vi "Emerson 5700 Example.vi"(8 "Error In":errorcluster, 10 "Remote Port":u16=502, 11 "Remote IP Address":string="10.2.0.49") -> (0 "Error Out":errorcluster, 3 "Emerson Flow Meter Data Output":T2={"Mass Flow Rate (Scaled Integer)"=0, "Density (Scaled Integer)"=8, "Temperature (Scaled Integer)"=114, "Volume Flow Rate (Scaled Integer)"=0, "Totalizer 1 (Scaled Integer)"=5, "Totalizer 2 (Scaled Integer)"=0, "Transmitter Software Rev"=14, "Flow Direction"="Forward", "Mass Flow Units"="lb/min", "Density Units"="lb/US Gal", "Temperature Units"="°F", "Volume Flow Units"="US GPM", "Pressure Units"="PSI", "Mass Total Units"="lbs", "Volume Total Units"="US Gallon", "Inventory 1 (Scaled Integer)"=5, "Inventory 2 (Scaled Integer)"=0, "Mass Flow Rate"=0.0, "Density"=8.2493896484375, "Temperature"=114.62187957763672, "Volume Flow Rate"=0.0, "Pressure (Scaled Integer)"=0, "Current Value Totalizer 1 (Pounds per draw)"=5.467781066894531, "Current Value Totalizer 2 (Gallons per draw)"=0.6632421612739563, "Current Value Inventory 1 (Pounds Total)"=5.467781066894531, "Current Value Inventory 2 (Gallons Total)"=0.6632421612739563, "Drive Gain"=7.360586643218994, "Raw Tube Frequency (Hz)"=151.36962890625, "Dynamic Viscosity (Centipoise)"=0.0, "Kinematic Viscosity (Centistokes)"=0.0, "Hot Gallons (Calculated Gallons)"=0.0, "Hot Flow Rate (Calculated GPM)"=0.0, "Hot Gallons Inventory (Gallons)"=0.0, "Hot Flow Rate (Laurel)"=0.0, "Hot Gallons (Laurel)"=0.0})   [LabVIEW 2019]
uses:
  Type Definitions/Emerson 5700 Data.ctl
  Type Definitions/Emerson 5700 Modbus Write Coils.ctl
  <vilib>/NI/Modbus Library/API/Master/Modbus Master.lvclass
  <vilib>/NI/Modbus Library/API/Wrapper/Create TCP Master.vi
  <vilib>/NI/Modbus Library/API/Wrapper/API Main.lvlib
panel:
  in  "address":string
  in  "Start/Stop Inventory 2.":T1=368 items=["Start/Stop Inventory 1"=367, "Start/Stop Inventory 2"=368, "Start/Stop all Totalizers and Inventories"=2, "Reset all Totalizers"=3, "Reset all Inventories"=4, "Reset Totalizer 1"=56, "Reset Totalizer 2"=57]
  in  "Start/Stop Inventory 1.":T1=367 items=["Start/Stop Inventory 1"=367, "Start/Stop Inventory 2"=368, "Start/Stop all Totalizers and Inventories"=2, "Reset all Totalizers"=3, "Reset all Inventories"=4, "Reset Totalizer 1"=56, "Reset Totalizer 2"=57]
  in  "Start/Stop Inventory 1":bool
  in  "Start/Stop Inventory 2":bool
  in  "Start/Stop all Totalizers and Inventories":bool
  in  "Reset all Totalizers":bool
  in  "Reset all Inventories":bool
  in  "Start/Stop all Totalizers and Inventories.":T1=2 items=["Start/Stop Inventory 1"=367, "Start/Stop Inventory 2"=368, "Start/Stop all Totalizers and Inventories"=2, "Reset all Totalizers"=3, "Reset all Inventories"=4, "Reset Totalizer 1"=56, "Reset Totalizer 2"=57]
  in  "Reset all Totalizers.":T1=3 items=["Start/Stop Inventory 1"=367, "Start/Stop Inventory 2"=368, "Start/Stop all Totalizers and Inventories"=2, "Reset all Totalizers"=3, "Reset all Inventories"=4, "Reset Totalizer 1"=56, "Reset Totalizer 2"=57]
  in  "Reset all Inventories.":T1=4 items=["Start/Stop Inventory 1"=367, "Start/Stop Inventory 2"=368, "Start/Stop all Totalizers and Inventories"=2, "Reset all Totalizers"=3, "Reset all Inventories"=4, "Reset Totalizer 1"=56, "Reset Totalizer 2"=57]
  in  "Reset Totalizer 2.":T1=57 items=["Start/Stop Inventory 1"=367, "Start/Stop Inventory 2"=368, "Start/Stop all Totalizers and Inventories"=2, "Reset all Totalizers"=3, "Reset all Inventories"=4, "Reset Totalizer 1"=56, "Reset Totalizer 2"=57]
  in  "Reset Totalizer 1.":T1=56 items=["Start/Stop Inventory 1"=367, "Start/Stop Inventory 2"=368, "Start/Stop all Totalizers and Inventories"=2, "Reset all Totalizers"=3, "Reset all Inventories"=4, "Reset Totalizer 1"=56, "Reset Totalizer 2"=57]
  in  "Reset Totalizer 2":bool
  in  "Reset Totalizer 1":bool
  in  "Emerson Flow Meter Data Input":T2
  # "Send Commands"
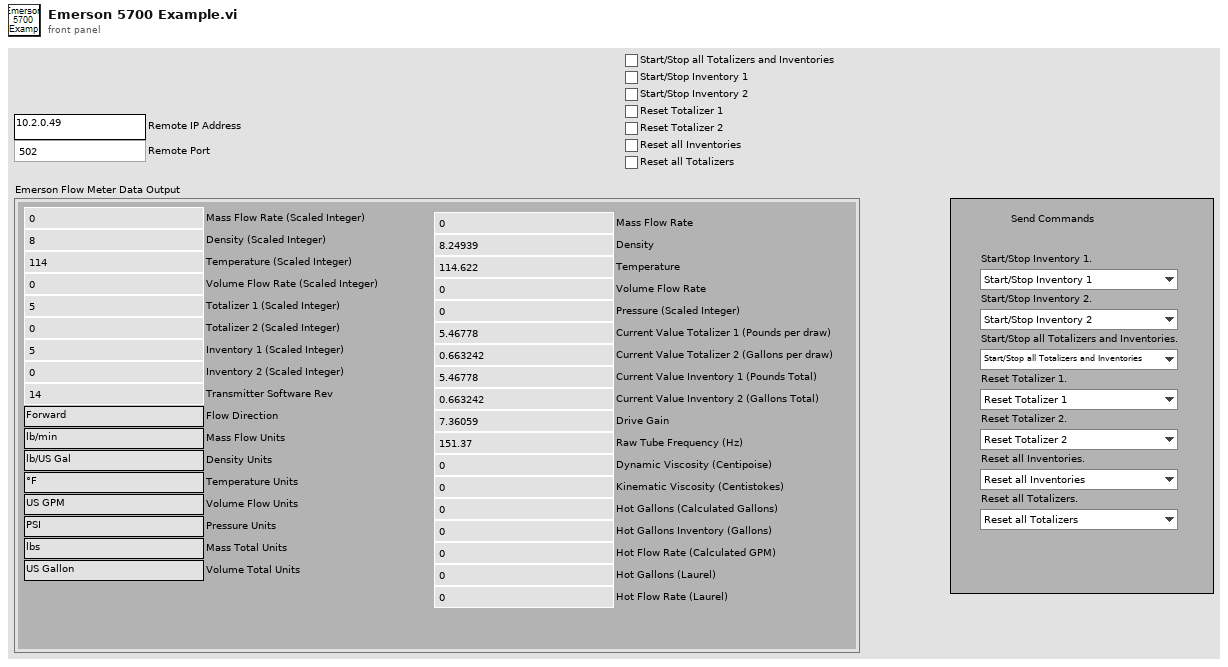
[diagram p1: front panel]
types:
  T1 = typedef "Emerson 5700 Modbus Write Coils.ctl" = u16
  T2 = typedef "Emerson 5700 Data.ctl" = cluster{"Mass Flow Rate (Scaled Integer)":u16, "Density (Scaled Integer)":u16, "Temperature (Scaled Integer)":u16, "Volume Flow Rate (Scaled Integer)":u16, "Totalizer 1 (Scaled Integer)":u16, "Totalizer 2 (Scaled Integer)":u16, "Transmitter Software Rev":u16, "Flow Direction":string, "Mass Flow Units":string, "Density Units":string, "Temperature Units":string, "Volume Flow Units":string, "Pressure Units":string, "Mass Total Units":string, "Volume Total Units":string, "Inventory 1 (Scaled Integer)":u16, "Inventory 2 (Scaled Integer)":u16, "Mass Flow Rate":dbl, "Density":dbl, "Temperature":dbl, "Volume Flow Rate":dbl, "Pressure (Scaled Integer)":u16, "Current Value Totalizer 1 (Pounds per draw)":dbl, "Current Value Totalizer 2 (Gallons per draw)":dbl, "Current Value Inventory 1 (Pounds Total)":dbl, "Current Value Inventory 2 (Gallons Total)":dbl, "Drive Gain":dbl, "Raw Tube Frequency (Hz)":dbl, "Dynamic Viscosity (Centipoise)":dbl, "Kinematic Viscosity (Centistokes)":dbl, "Hot Gallons (Calculated Gallons)":dbl, "Hot Flow Rate (Calculated GPM)":dbl, "Hot Gallons Inventory (Gallons)":dbl, "Hot Flow Rate (Laurel)":dbl, "Hot Gallons (Laurel)":dbl}
  T3 = enum32{"invalid app kind", "Development System", "Run Time System", "Student Edition", "Embedded LabVIEW", "Evaluation", "Custom"}
  T4 = enum32{"Invalid", "Standard", "Closed", "Hidden", "Minimized", "Maximized"}
  T5 = cluster{"Core":cluster{"Current VI Reference":refnum<vi>, "Close Panel on Exit?":bool}, "Remote IP Address":string, "Remote Port":u16, "TCP master instance":refnum<class "Modbus Master.lvclass">, "Emerson Flow Meter Data Input":T2}
  T6 = cluster{"Current VI Reference":refnum<vi>, "Close Panel on Exit?":bool}
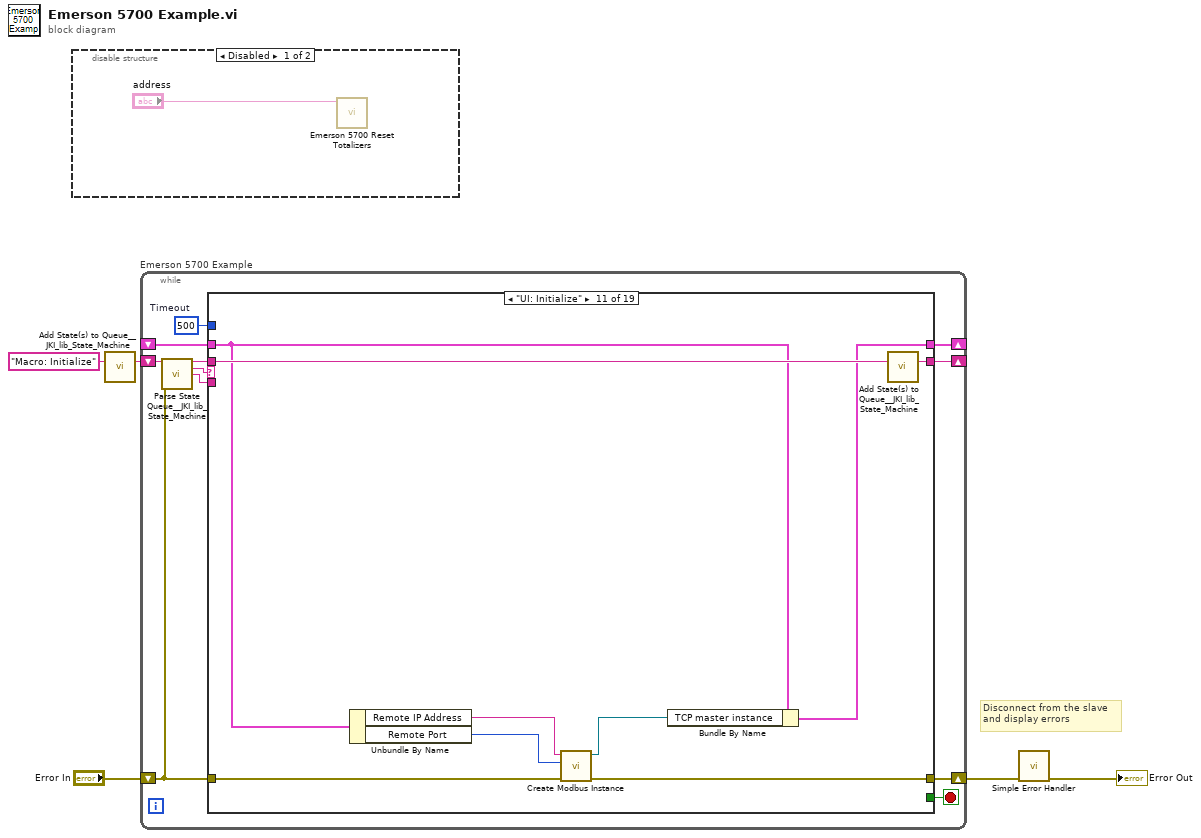
[diagram p0: block diagram]
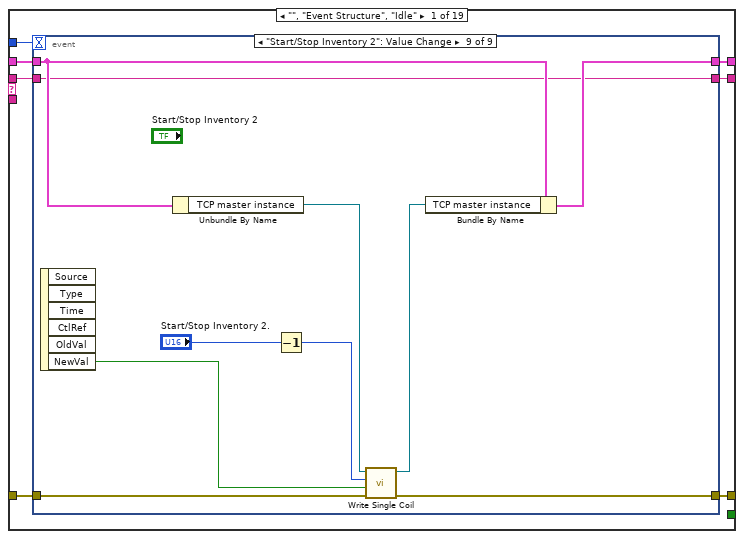
[diagram p3: hidden frame]
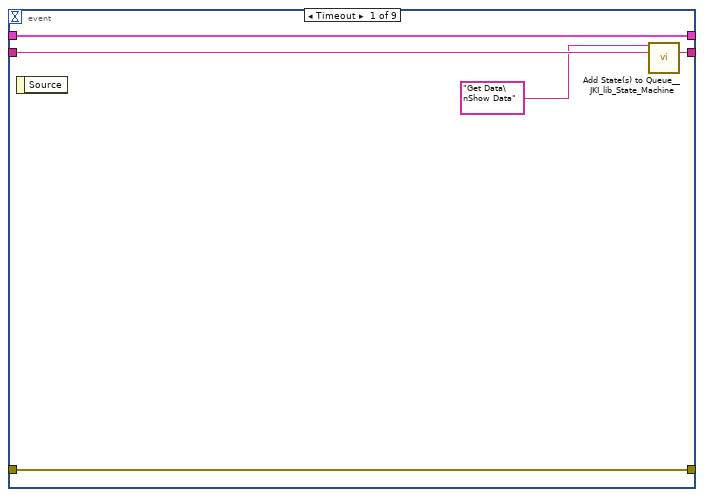
[diagram p4: hidden frame]
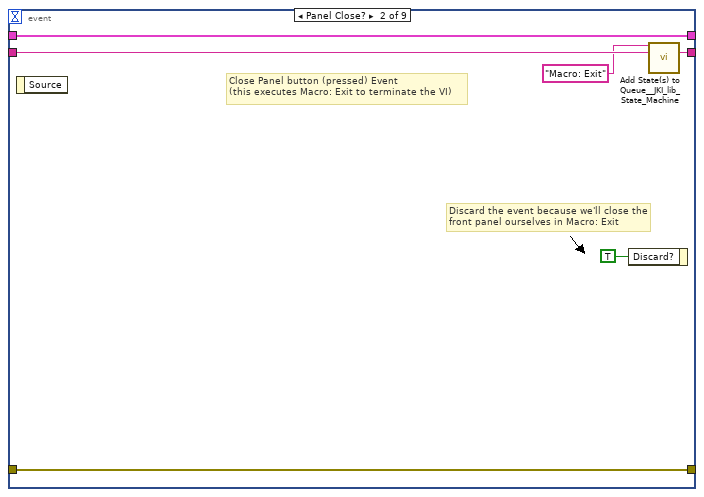
[diagram p5: hidden frame]
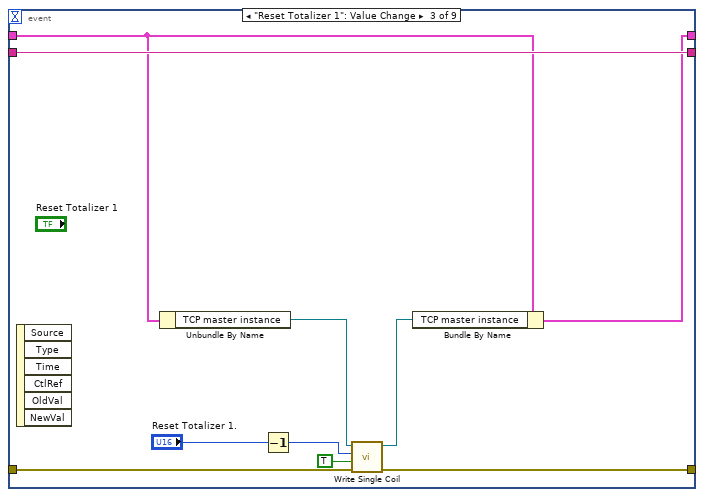
[diagram p6: hidden frame]
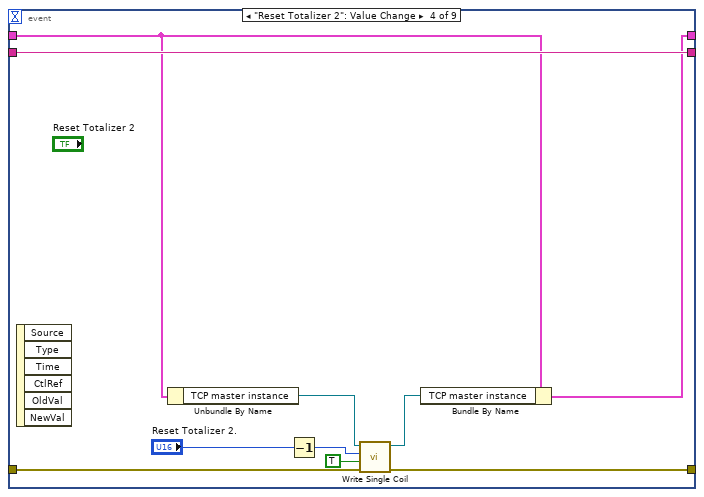
[diagram p7: hidden frame]
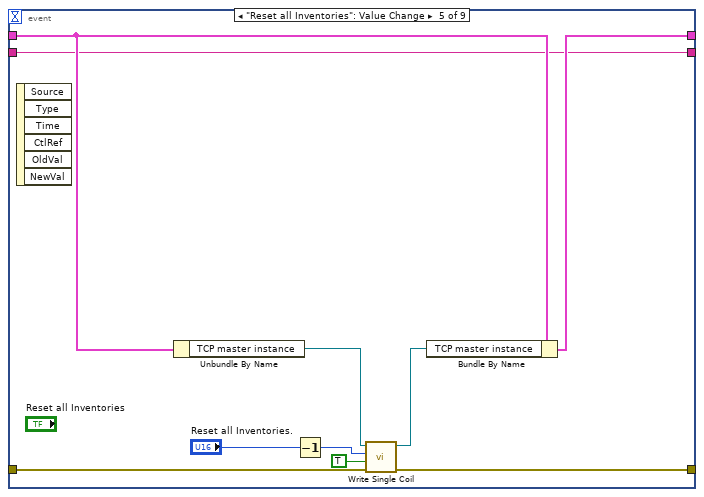
[diagram p8: hidden frame]
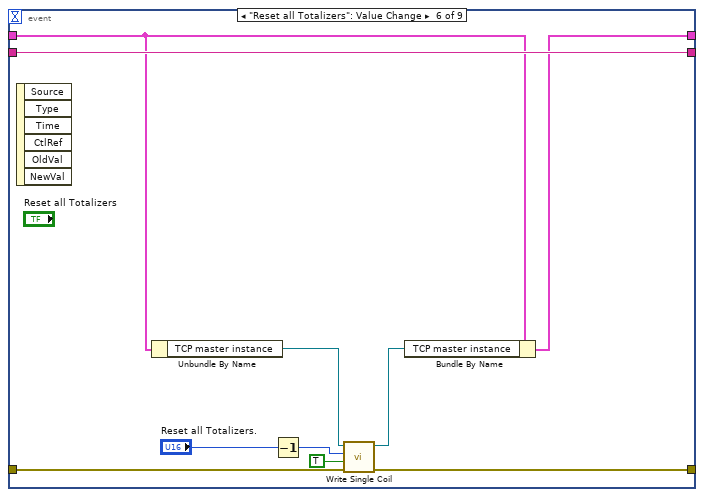
[diagram p9: hidden frame]
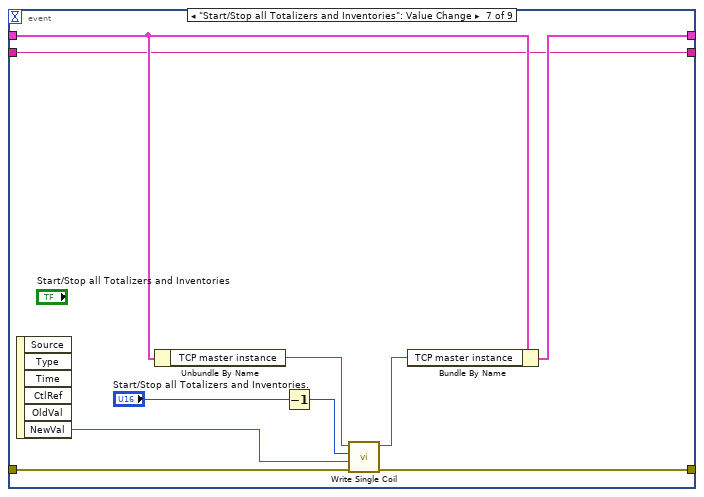
[diagram p10: hidden frame]
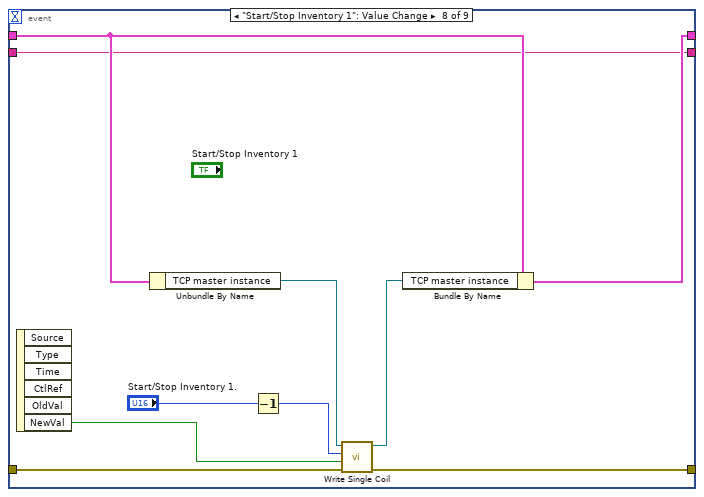
[diagram p11: hidden frame]
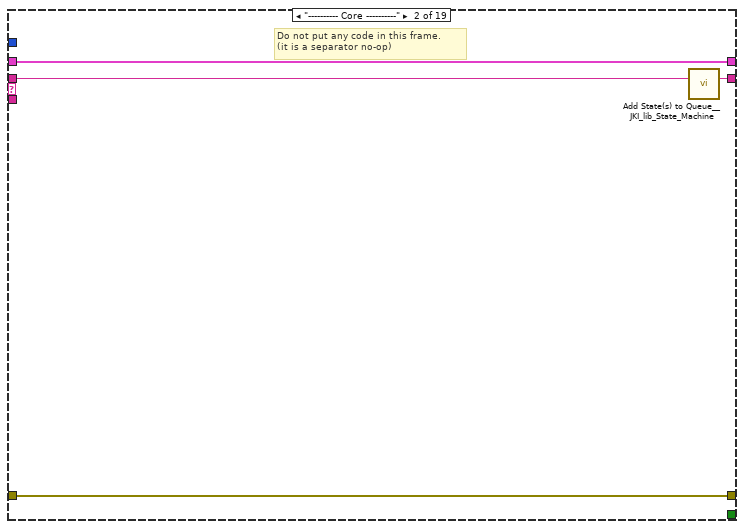
[diagram p12: hidden frame]
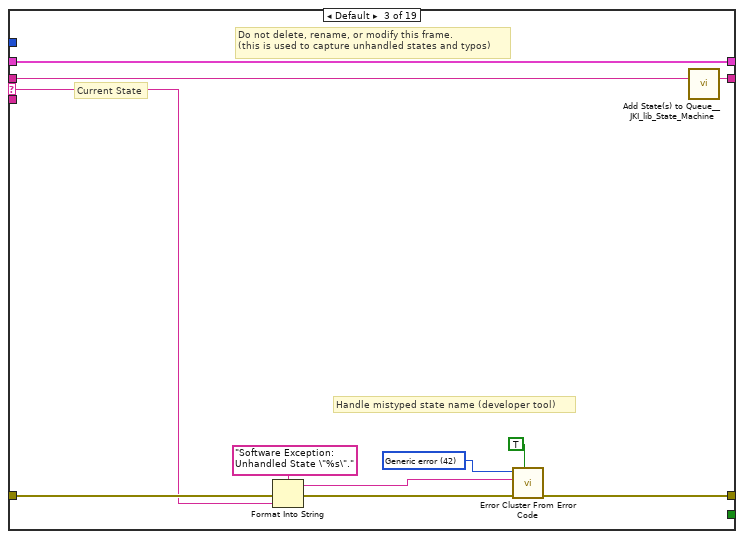
[diagram p13: hidden frame]
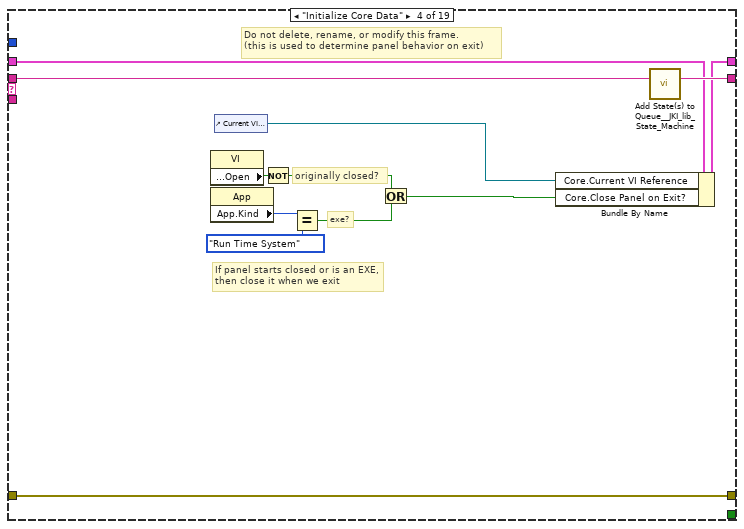
[diagram p14: hidden frame]
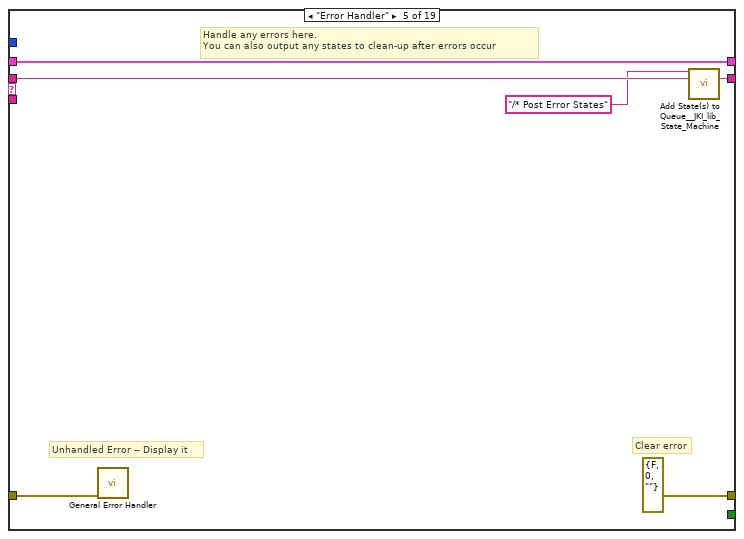
[diagram p15: hidden frame]
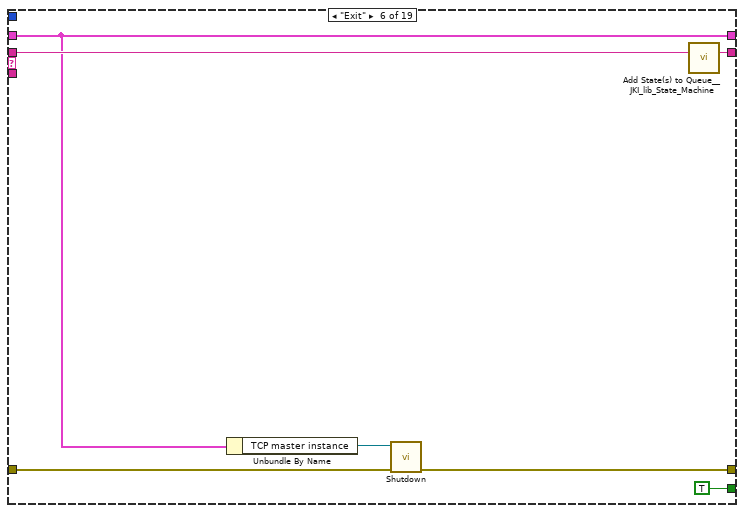
[diagram p16: hidden frame]
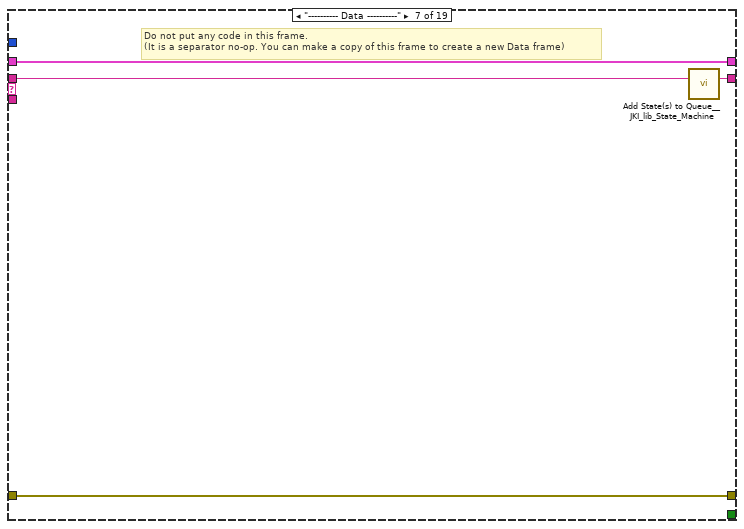
[diagram p17: hidden frame]
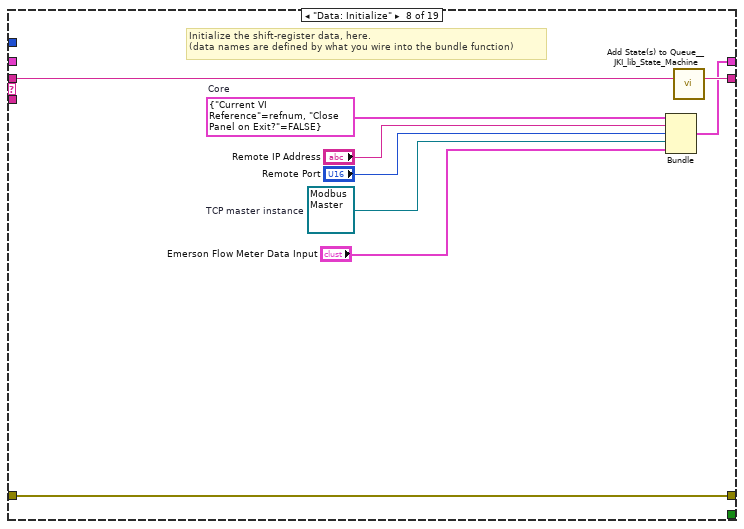
[diagram p18: hidden frame]
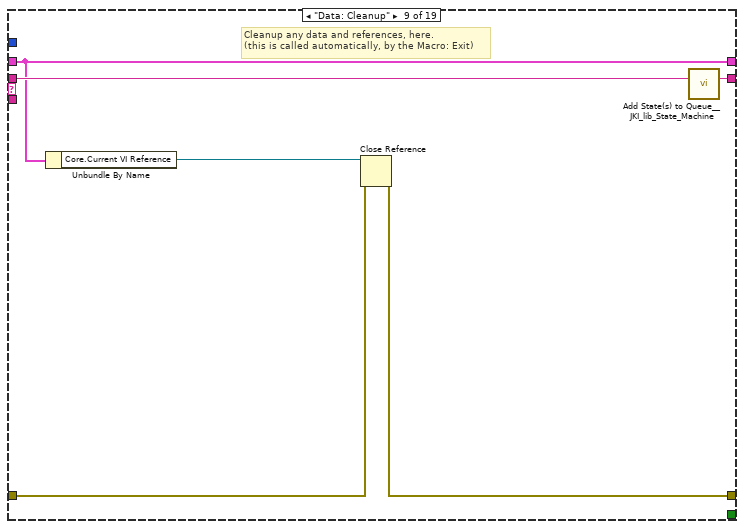
[diagram p19: hidden frame]
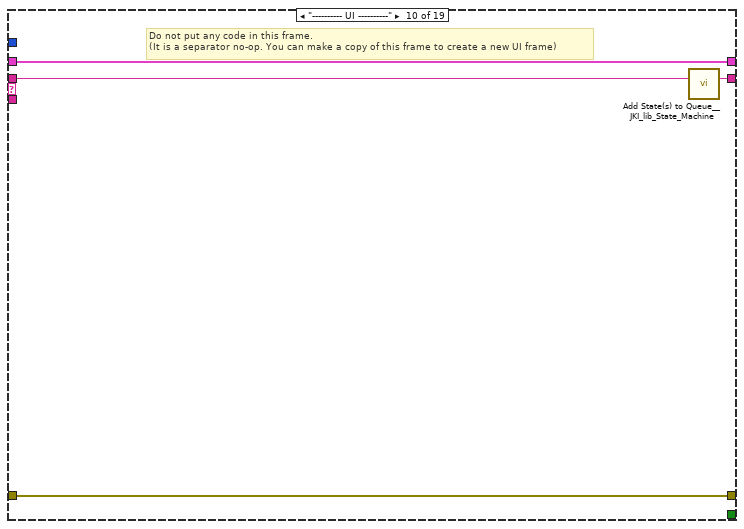
[diagram p20: hidden frame]
diagram:
  # "Disconnect from the slave\nand display errors"
  n1 = disable-structure shown="Disabled" {
    frame Disabled {
      n2 = call "Emerson 5700 Reset Totalizers.vi"("address"="address") -> ()  [unwired: 10 in, 1 out]
    }
    frame Enabled {
    }
  }
  n3 = call <vilib>:"Add State(s) to Queue__JKI_lib_State_Machine.vi"("State(s) in (\"\")"="Macro: Initialize") -> ("States Out"=w5:string)  [unwired: 14 in]
  n4 = while "Emerson 5700 Example" {
    shift-right: [w10] -> _
    shift-left: _ -> [w9]
    shift-right: [w13] -> w2
    shift-left: "Error In" -> [w7]
    shift-right: [w12] -> _
    shift-left: w5 -> [w14]
    stop <- w11 stop-if-true
    w8 = 500  # Timeout
    n5 = call <vilib>:"Parse State Queue__JKI_lib_State_Machine.vi"("State Queue"=w14, "Error In (no error)"=w7) -> ("Remaining States"=w16:string, "Current State"=w17:string, "Arguments"=w15:string)  [unwired: 11 in]
    n6 = case shown="\"UI: Initialize\"" w17 {
      selector: w17 -> [_ _ w110 _ _ _ _ _ _ _ _ _ _ _ _ _ _ _ _]
      tunnel: w16 -> [w24 w109 w114 w132 w138 w145 w149 w158 w164 w168 w177 w183 w194 w220 w225 w235 w239 w252 w257]
      tunnel: w15 -> [_ _ _ _ _ _ _ _ _ _ _ w178 w188 _ _ _ _ _ _]
      tunnel: w9 -> [w22 w106 w112 w123 w135 w140 w146 _ w159 w165 w171 w181 w190 w217 w222 w232 w236 w243 w254]
      tunnel: [w21 w107 w116 w129 errorcluster {"status"=FALSE, "code"=0, "source"=""} ("error out") w141 w147 w155 w160 w166 w174 w179 w191 w218 w223 w233 w237 w246 w255] -> w13
      tunnel: w7 -> [w20 w107 w115 w129 w134 w142 w147 w155 w161 w166 w175 w180 w192 w218 w223 w233 w237 w247 w255]
      tunnel: [w23 w108 w113 w131 w137 w144 w148 w157 w163 w167 w176 w182 w193 w219 w224 w234 w238 w251 w256] -> w12
      tunnel: [_ _ _ _ _ TRUE _ _ _ _ _ _ _ _ _ _ _ _ _] -> w11
      tunnel: [w19 w106 w112 w130 w135 w140 w146 w156 w159 w165 w170 w181 w190 w217 w222 w232 w236 w242 w254] -> w10
      tunnel: w8 -> [w18 _ _ _ _ _ _ _ _ _ _ _ _ _ _ _ _ _ _]
      frame "", "Event Structure", "Idle" {
        n7 = event shown="[8] \"Start/Stop Inventory 2\": Value Change" {
          selector: _ -> [_ _ _ _ _ _ _ _ _]
          dyn-events: _ -> [_ _ _ _ _ _ _ _ _]
          timeout: w18 -> [_ _ _ _ _ _ _ _ _]
          tunnel: w24 -> [w29 w35 w42 w50 w58 w68 w77 w90 w98]
          tunnel: [w28 w34 w42 w50 w58 w68 w77 w90 w98] -> w23
          tunnel: w22 -> [w26 w32 w40 w49 w59 w67 w78 w92 w100]
          tunnel: [w27 w33 w43 w51 w56 w70 w81 w86 w101] -> w21
          tunnel: w20 -> [w27 w33 w44 w52 w57 w71 w82 w87 w102]
          tunnel: [w26 w32 w39 w48 w60 w66 w79 w91 w99] -> w19
          event Timeout {
            n8 = event-data() -> ()  [unwired: 1 in, 1 out]
            n9 = call <vilib>:"Add State(s) to Queue__JKI_lib_State_Machine.vi"("State(s) in Front (\"\")"="Get Data\nShow Data" ("State(s) in Front (\"\")"), "State(s) in (\"\")"=w29) -> ("States Out"=w28:string)  [unwired: 13 in]
          }
          event Panel Close? {
            # "Discard the event because we'll close the front panel ourselves in Macro: Exit"
            # "Close Panel button (pressed) Event\n(this executes Macro: Exit to terminate the VI)"
            n10 = event-data() -> ()  [unwired: 1 in, 1 out]
            n11 = event-data("Discard?"=TRUE) -> ()  [unwired: 1 in, 1 out]
            n12 = call <vilib>:"Add State(s) to Queue__JKI_lib_State_Machine.vi"("State(s) in Front (\"\")"="Macro: Exit", "State(s) in (\"\")"=w35) -> ("States Out"=w34:string)  [unwired: 13 in]
          }
          event "Reset Totalizer 1": Value Change {
            n13 = event-data() -> ()  [unwired: 1 in, 6 out]
            n14 = Unbundle By Name(w40) -> ("TCP master instance"=w41:refnum<class "Modbus Master.lvclass">)
            n15 = Decrement(x="Reset Totalizer 1.") -> (x-1=w37:T1)
            n16 = call-dynamic "Write Single Coil.vi"("error in"=w44, "coil to write"=TRUE ("Coil"), "address"=w37, "Modbus master in"=w41) -> ("error out"=w43:errorcluster, "Modbus master out"=w38:refnum<class "Modbus Master.lvclass">)  [unwired: 6 in]
            n17 = Bundle By Name(cluster=w40, "TCP master instance"=w38) -> (w39:T5)
          }
          event "Reset Totalizer 2": Value Change {
            n18 = event-data() -> ()  [unwired: 1 in, 6 out]
            n19 = Unbundle By Name(w49) -> ("TCP master instance"=w54:refnum<class "Modbus Master.lvclass">)
            n20 = Decrement(x="Reset Totalizer 2.") -> (x-1=w47:T1)
            n21 = call-dynamic "Write Single Coil.vi"("error in"=w52, "coil to write"=TRUE ("Coil"), "address"=w47, "Modbus master in"=w54) -> ("error out"=w51:errorcluster, "Modbus master out"=w53:refnum<class "Modbus Master.lvclass">)  [unwired: 6 in]
            n22 = Bundle By Name(cluster=w49, "TCP master instance"=w53) -> (w48:T5)
          }
          event "Reset all Inventories": Value Change {
            n23 = event-data() -> ()  [unwired: 1 in, 6 out]
            n24 = Unbundle By Name(w59) -> ("TCP master instance"=w64:refnum<class "Modbus Master.lvclass">)
            n25 = Decrement(x="Reset all Inventories.") -> (x-1=w62:T1)
            n26 = call-dynamic "Write Single Coil.vi"("error in"=w57, "coil to write"=TRUE ("Coil"), "address"=w62, "Modbus master in"=w64) -> ("error out"=w56:errorcluster, "Modbus master out"=w63:refnum<class "Modbus Master.lvclass">)  [unwired: 6 in]
            n27 = Bundle By Name(cluster=w59, "TCP master instance"=w63) -> (w60:T5)
          }
          event "Reset all Totalizers": Value Change {
            n28 = event-data() -> ()  [unwired: 1 in, 6 out]
            n29 = Unbundle By Name(w67) -> ("TCP master instance"=w74:refnum<class "Modbus Master.lvclass">)
            n30 = Decrement(x="Reset all Totalizers.") -> (x-1=w72:T1)
            n31 = call-dynamic "Write Single Coil.vi"("error in"=w71, "coil to write"=TRUE ("Coil"), "address"=w72, "Modbus master in"=w74) -> ("error out"=w70:errorcluster, "Modbus master out"=w73:refnum<class "Modbus Master.lvclass">)  [unwired: 6 in]
            n32 = Bundle By Name(cluster=w67, "TCP master instance"=w73) -> (w66:T5)
          }
          event "Start/Stop all Totalizers and Inventories": Value Change {
            n33 = event-data() -> ("NewVal"=w76:bool)  [unwired: 1 in, 5 out]
            n34 = Unbundle By Name(w78) -> ("TCP master instance"=w85:refnum<class "Modbus Master.lvclass">)
            n35 = Decrement(x="Start/Stop all Totalizers and Inventories.") -> (x-1=w83:T1)
            n36 = call-dynamic "Write Single Coil.vi"("error in"=w82, "coil to write"=w76, "address"=w83, "Modbus master in"=w85) -> ("error out"=w81:errorcluster, "Modbus master out"=w84:refnum<class "Modbus Master.lvclass">)  [unwired: 6 in]
            n37 = Bundle By Name(cluster=w78, "TCP master instance"=w84) -> (w79:T5)
          }
          event "Start/Stop Inventory 1": Value Change {
            n38 = event-data() -> ("NewVal"=w89:bool)  [unwired: 1 in, 5 out]
            n39 = Unbundle By Name(w92) -> ("TCP master instance"=w95:refnum<class "Modbus Master.lvclass">)
            n40 = Decrement(x="Start/Stop Inventory 1.") -> (x-1=w93:T1)
            n41 = call-dynamic "Write Single Coil.vi"("error in"=w87, "coil to write"=w89, "address"=w93, "Modbus master in"=w95) -> ("error out"=w86:errorcluster, "Modbus master out"=w94:refnum<class "Modbus Master.lvclass">)  [unwired: 6 in]
            n42 = Bundle By Name(cluster=w92, "TCP master instance"=w94) -> (w91:T5)
          }
          event "Start/Stop Inventory 2": Value Change {
            n43 = event-data() -> ("NewVal"=w96:bool)  [unwired: 1 in, 5 out]
            n44 = Unbundle By Name(w100) -> ("TCP master instance"=w105:refnum<class "Modbus Master.lvclass">)
            n45 = Decrement(x="Start/Stop Inventory 2.") -> (x-1=w103:T1)
            n46 = call-dynamic "Write Single Coil.vi"("error in"=w102, "coil to write"=w96, "address"=w103, "Modbus master in"=w105) -> ("error out"=w101:errorcluster, "Modbus master out"=w104:refnum<class "Modbus Master.lvclass">)  [unwired: 6 in]
            n47 = Bundle By Name(cluster=w100, "TCP master instance"=w104) -> (w99:T5)
          }
        }
      }
      frame "---------- Core ----------" {
        # "Do not put any code in this frame.\n(it is a separator no-op)"
        n48 = call <vilib>:"Add State(s) to Queue__JKI_lib_State_Machine.vi"("State(s) in (\"\")"=w109) -> ("States Out"=w108:string)  [unwired: 14 in]
      }
      frame Default {
        w119 = 42 items=["No error", "Argument error", "Memory is full", "Out of zone", "End of file", "File already open", "Generic file I/O error", "File not found", "File permission error", "Disk is full", "Duplicate path", "Too many files open", "System feature not enabled", "Resource file not found", "Cannot add resource", "Resource not found", "Image not found", "Image memory error", "Pen does not exist", "Config type invalid", "Config token not found", "Config parse error", "Config memory error", "Bad external code format", "Bad external code offset", "External code not present", "Null window", "Destroy window error", "Null menu", "Print aborted", "Bad print record", "Print driver error", "Windows error during printing", "Memory error during printing", "Print dialog error", "Generic print error", "Invalid device refnum", "Device not found", "Device parameter error", "Device unit error", "Cannot open device", "Device call aborted", "Generic error", "Cancelled by user", "Object ID too low", "Object ID too high", "Object not in heap", "Unknown heap", "Unknown object (invalid DefProc)", "Unknown object (DefProc not in table)", "Message out of range", "Invalid (null) method", "Unknown message", "Manager call not supported", "Bad address", "Network operation in progress", "Network operation timed out", "Connection is busy", "Network attribute not supported", "Network error", "Address in use", "System out of memory", "Connection aborted", "Connection refused", "Not connected", "Already connected", "Connection closed", "Initialization error (interapplication manager)", "Bad occurrence", "Wait on unbound occurrence handler", "Occurrence queue overflow", "Datalog type conflict", "Unused", "Unrecognized type (interapplication manager)", "Memory corrupt", "Failed to make temporary DLL", "Old CIN version", "Drag socket not found", "Failed to load drop-object", "Failed to register OLE object", "Failed to release OLE object", "Format specifier type mismatch", "Unknown format specifier", "Too few format specifiers", "Too many format specifiers", "Scan failed", "Newer CIN version", "Error converting to variant", "Runtime menu error", "Password tampered", "Variant attribute not found", "Incompatible variant data type", "Event data is not available", "Event Store is not present", "Occurrence is not found", "Event Queue is not created", "Event info is not available", "Refnum passed is NULL", "Error retrieving Class GUID", "Error retrieving CoClass GUID", "Error retrieving TypeLib GUID.", "Bad built application magic bytes.", "Specific driver is different from the specific driver associated with the Logical Name.", "There is no session opened to the class driver.", "Max Error", "MAX - Error with config objects", "MAX - Error loading configuration", "MAX - Group not supported"]
        # "Current State"
        # "Do not delete, rename, or modify this frame.\n(this is used to capture unhandled states and typos)"
        # "Handle mistyped state name (developer tool)"
        n49 = Format Into String(format string="Software Exception: Unhandled State \"%s\"." ("message"), error in=w115, w110) -> (resulting string=w118:string, error out=w117:errorcluster)  [unwired: 1 in]
        n50 = call <vilib>:"Error Cluster From Error Code.vi"("show call chain? (False)"=TRUE, "error in (no error)"=w117, "error message (\"\")"=w118, "error code (0)"=w119) -> ("error out"=w116:errorcluster)  [unwired: 5 in]
        n51 = call <vilib>:"Add State(s) to Queue__JKI_lib_State_Machine.vi"("State(s) in (\"\")"=w114) -> ("States Out"=w113:string)  [unwired: 14 in]
      }
      frame "Initialize Core Data" {
        # "Do not delete, rename, or modify this frame.\n(this is used to determine panel behavior on exit)"
        # "originally closed?"
        # "exe?"
        # "If panel starts closed or is an EXE, then close it when we exit"
        n52 = property class="VI"() -> ("Front Panel.Open"=w128:bool)  [unwired: 2 in, 2 out]
        n53 = property class="App"() -> ("App.Kind"=w127:T3)  [unwired: 2 in, 2 out]
        n54 = control-ref of="Current VI Reference"() -> (w121:refnum<vi>)
        n55 = Not(x=w128) -> (.not. x?=w125:bool)
        n56 = Equal?(x=w127, y=T3."Run Time System" ("Application:Kind")) -> (x = y?=w124:bool)
        n57 = Or(x=w125, y=w124) -> (x .or. y?=w122:bool)
        n58 = Bundle By Name(cluster=w123, "Core.Current VI Reference"=w121, "Core.Close Panel on Exit?"=w122) -> (w130:T5)
        n59 = call <vilib>:"Add State(s) to Queue__JKI_lib_State_Machine.vi"("State(s) in (\"\")"=w132) -> ("States Out"=w131:string)  [unwired: 14 in]
      }
      frame "Error Handler" {
        # "Unhandled Error -- Display it"
        # "Handle any errors here.\nYou can also output any states to clean-up after errors occur"
        # "Clear error"
        n60 = call <vilib>:"General Error Handler.vi"("error in (no error)"=w134) -> ()  [unwired: 10 in, 5 out]
        n61 = call <vilib>:"Add State(s) to Queue__JKI_lib_State_Machine.vi"("State(s) in Front (\"\")"="/* Post Error States", "State(s) in (\"\")"=w138) -> ("States Out"=w137:string)  [unwired: 13 in]
      }
      frame "Exit" {
        n62 = Unbundle By Name(w140) -> ("TCP master instance"=w139:refnum<class "Modbus Master.lvclass">)
        n63 = call-dynamic "Shutdown.vi"("error in"=w142, "Modbus master in"=w139) -> ("error out"=w141:errorcluster)  [unwired: 9 in]
        n64 = call <vilib>:"Add State(s) to Queue__JKI_lib_State_Machine.vi"("State(s) in (\"\")"=w145) -> ("States Out"=w144:string)  [unwired: 14 in]
      }
      frame "---------- Data ----------" {
        # "Do not put any code in this frame.\n(It is a separator no-op. You can make a copy of this frame to create a new Data frame)"
        n65 = call <vilib>:"Add State(s) to Queue__JKI_lib_State_Machine.vi"("State(s) in (\"\")"=w149) -> ("States Out"=w148:string)  [unwired: 14 in]
      }
      frame "Data: Initialize" {
        w151 = refnum<class "Modbus Master.lvclass"> refnum  # TCP master instance
        w154 = T6 {"Current VI Reference"=refnum, "Close Panel on Exit?"=FALSE}  # Core
        # "Initialize the shift-register data, here.\n(data names are defined by what you wire into the bundle function)"
        n66 = Bundle("Core"=w154, "Remote IP Address"="Remote IP Address", "Remote Port"="Remote Port", "TCP master instance"=w151, "Emerson Flow Meter Data Input"="Emerson Flow Meter Data Input") -> (w156:T5)  [unwired: 1 in]
        n67 = call <vilib>:"Add State(s) to Queue__JKI_lib_State_Machine.vi"("State(s) in (\"\")"=w158) -> ("States Out"=w157:string)  [unwired: 14 in]
      }
      frame "Data: Cleanup" {
        # "Cleanup any data and references, here.\n(this is called automatically, by the Macro: Exit)"
        n68 = Unbundle By Name(w159) -> ("Core.Current VI Reference"=w162:refnum<vi>)
        n69 = Close Reference(reference=w162, error in (no error)=w161) -> (error out=w160:errorcluster)
        n70 = call <vilib>:"Add State(s) to Queue__JKI_lib_State_Machine.vi"("State(s) in (\"\")"=w164) -> ("States Out"=w163:string)  [unwired: 14 in]
      }
      frame "---------- UI ----------" {
        # "Do not put any code in this frame.\n(It is a separator no-op. You can make a copy of this frame to create a new UI frame)"
        n71 = call <vilib>:"Add State(s) to Queue__JKI_lib_State_Machine.vi"("State(s) in (\"\")"=w168) -> ("States Out"=w167:string)  [unwired: 14 in]
      }
      frame "UI: Initialize" {
        n72 = Unbundle By Name(w171) -> ("Remote IP Address"=w173:string, "Remote Port"=w172:u16)
        n73 = call-poly <vilib>:"Create Modbus Instance.vi"("error in"=w175, "port (502)"=w172, "address"=w173) -> ("error out"=w174:errorcluster, "TCP master instance"=w169:refnum<class "Modbus Master.lvclass">)  [unwired: 7 in]
        n74 = Bundle By Name(cluster=w171, "TCP master instance"=w169) -> (w170:T5)
        n75 = call <vilib>:"Add State(s) to Queue__JKI_lib_State_Machine.vi"("State(s) in (\"\")"=w177) -> ("States Out"=w176:string)  [unwired: 14 in]
      }
      frame "UI: Cursor Set" {
        # "Argument"
        # "Set and Unset Cursor Busy.\n(Usage: \"UI: Cursor Set >> Busy|Idle\")"
        n76 = case shown="\"Idle\", Default" w178 {
          tunnel: w180 -> [w185 w187]
          tunnel: [w184 w186] -> w179
          frame "Idle", Default {
            n77 = call <vilib>:"Unset Busy.vi"("error in (no error)"=w185) -> ("error out"=w184:errorcluster)  [unwired: 10 in]
          }
          frame "Busy" {
            n78 = call <vilib>:"Set Busy.vi"("error in (no error)"=w187) -> ("error out"=w186:errorcluster)  [unwired: 9 in, 1 out]
          }
        }
        n79 = call <vilib>:"Add State(s) to Queue__JKI_lib_State_Machine.vi"("State(s) in (\"\")"=w183) -> ("States Out"=w182:string)  [unwired: 14 in]
      }
      frame "UI: Front Panel State" {
        # "Argument"
        # "Set Front Panel Open or Closed\n(Usage: \"UI: Front Panel State >> Open|Close\")"
        n80 = Unbundle By Name(w190) -> ("Core.Current VI Reference"=w189:refnum<vi>)
        n81 = case shown="\"Open\", Default" w188 {
          tunnel: w192 -> [w198 w211]
          tunnel: [w200 w212] -> w191
          tunnel: w189 -> [w199 w209]
          frame "Open", Default {
            n82 = property class="VI"(reference=w199, error in=w198) -> (reference out=w196:refnum<vi>, error out=w197:errorcluster, "Front Panel.Open"=w195:bool)
            n83 = case shown="False" w195 {
              tunnel: [w203 w206] -> w200
              tunnel: w197 -> [w202 w206]
              tunnel: w196 -> [w201 _]
              frame False {
                n84 = invoke class="VI" method="FP.Open"(reference=w201, error in=w202, "Activate"=TRUE, "State"=T4."Standard") -> (error out=w203:errorcluster)  [unwired: 1 in, 4 out]
              }
              frame True {
              }
            }
          }
          frame "Close" {
            n85 = property class="VI"(reference=w209, error in=w211) -> (reference out=w208:refnum<vi>, error out=w210:errorcluster, "Front Panel.Open"=w207:bool)
            n86 = case shown="True" w207 {
              tunnel: [w213 w216] -> w212
              tunnel: w210 -> [w213 w215]
              tunnel: w208 -> [_ w214]
              frame False {
              }
              frame True {
                n87 = invoke class="VI" method="FP.Close"(reference=w214, error in=w215) -> (error out=w216:errorcluster)  [unwired: 1 in, 2 out]
              }
            }
          }
        }
        n88 = call <vilib>:"Add State(s) to Queue__JKI_lib_State_Machine.vi"("State(s) in (\"\")"=w194) -> ("States Out"=w193:string)  [unwired: 14 in]
      }
      frame "---------- Macro ----------" {
        # "Do not put any code in this frame.\n(It is a separator no-op. You can make a copy of this frame to create a new Macro frame)"
        n89 = call <vilib>:"Add State(s) to Queue__JKI_lib_State_Machine.vi"("State(s) in (\"\")"=w220) -> ("States Out"=w219:string)  [unwired: 14 in]
      }
      frame "Macro: Initialize" {
        w221 = "Data: Initialize\nInitialize Core Data\nUI: Initialize\nUI: Front Panel State >> Open"  # Data: Initialize Initialize Core Data UI: Initialize UI: Front Panel State >> Open
        # "Initialization Macro\n(This is called once, when the VI starts)"
        n90 = call <vilib>:"Add State(s) to Queue__JKI_lib_State_Machine.vi"("State(s) in Front (\"\")"=w221, "State(s) in (\"\")"=w225) -> ("States Out"=w224:string)  [unwired: 13 in]
      }
      frame "Macro: Exit" {
        # "Exit Macro\n(This is called once, when the VI exits)"
        n91 = Unbundle By Name(w232) -> ("Core.Close Panel on Exit?"=w231:bool)
        n92 = Select(t="UI: Front Panel State >> Close", s=w231, f="") -> (s? t:f=w228:string)
        n93 = call <vilib>:"Add State(s) to Queue__JKI_lib_State_Machine.vi"("State(s) in (\"\")"=w228, "State(s) at Back (\"\")"="Data: Cleanup\nExit") -> ("States Out"=w226:string)  [unwired: 13 in]
        n94 = call <vilib>:"Add State(s) to Queue__JKI_lib_State_Machine.vi"("State(s) in Front (\"\")"=w226, "State(s) in (\"\")"=w235) -> ("States Out"=w234:string)  [unwired: 13 in]
      }
      frame "---------- New Category ----------" {
        # "Template Separator\n(You can make a copy of, or modify, this frame)"
        n95 = call <vilib>:"Add State(s) to Queue__JKI_lib_State_Machine.vi"("State(s) in (\"\")"=w239) -> ("States Out"=w238:string)  [unwired: 14 in]
      }
      frame "Get Data" {
        n96 = Unbundle By Name(w243) -> ("TCP master instance"=w245:refnum<class "Modbus Master.lvclass">, "Emerson Flow Meter Data Input"=w244:T2)
        n97 = call "Emerson 5700 16 Bit Data.vi"("error in (no error)"=w247, "Emerson Flow Meter Data Input"=w244, "Modbus Master in"=w245) -> ("error out"=w248:errorcluster, "Emerson Flow Meter Data Output"=w250:T2, "Modbus Master out"=w249:refnum<class "Modbus Master.lvclass">)  [unwired: 6 in]
        n98 = call "Emerson 5700 32 Bit Data.vi"("Error In"=w248, "Emerson Flow Meter Data Input"=w250, "Modbus master in"=w249) -> ("Error Out"=w246:errorcluster, "Emerson Flow Meter Data Output"=w240:T2, "Modbus master out"=w241:refnum<class "Modbus Master.lvclass">)  [unwired: 6 in]
        n99 = Bundle By Name(cluster=w243, "TCP master instance"=w241, "Emerson Flow Meter Data Input"=w240) -> (w242:T5)
        n100 = call <vilib>:"Add State(s) to Queue__JKI_lib_State_Machine.vi"("State(s) in (\"\")"=w252) -> ("States Out"=w251:string)  [unwired: 14 in]
      }
      frame "Show Data" {
        n101 = Unbundle By Name(w254) -> ("Emerson Flow Meter Data Input"=→"Emerson Flow Meter Data Output":T2)
        n102 = call <vilib>:"Add State(s) to Queue__JKI_lib_State_Machine.vi"("State(s) in (\"\")"=w257) -> ("States Out"=w256:string)  [unwired: 14 in]
      }
    }
  }
  n103 = call <vilib>:"Simple Error Handler.vi"("error in (no error)"=w2) -> ("error out"=→"Error Out":errorcluster)  [unwired: 1 in, 7 out]
